vi "UnpoweredState.vi"(8 "error in (no error)":errorcluster, 10 "Cluster in":T2, 11 "Enum in":T1) -> (0 "error out":errorcluster, 2 "Cluster out":T2, 3 "Enum":T1)   [LabVIEW 2018]
uses:
  Type_Def Actuator Controls.ctl
  Type_Def_Current_state_output.ctl
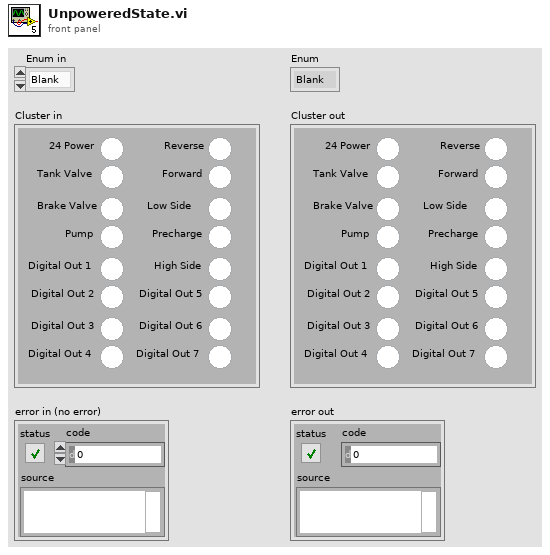
[diagram p1: front panel]
types:
  T1 = typedef "Type_Def_Current_state_output.ctl" = enum16{"Blank", "Systems Check", "Idle", "Ready", "Pushing", "CrawlingPrecharge", "Braking", "Fault", "Boot Up", "Unpowered", "Crawling", "Shutdown", "Service Push", "Service Wait", "Vent", "Precharge", "Cooldown"}
  T2 = typedef "Type_Def Actuator Controls.ctl" = cluster{"Reverse ":bool, "Forward":bool, "Low Side":bool, "Precharge":bool, "High Side":bool, "Digital Out 5":bool, "Digital Out 6":bool, "Digital Out 7 ":bool, "24 Power":bool, "Tank Valve ":bool, "Brake Valve":bool, "Pump":bool, "Digital Out 1 ":bool, "Digital Out 2":bool, "Digital Out 3":bool, "Digital Out 4 ":bool}
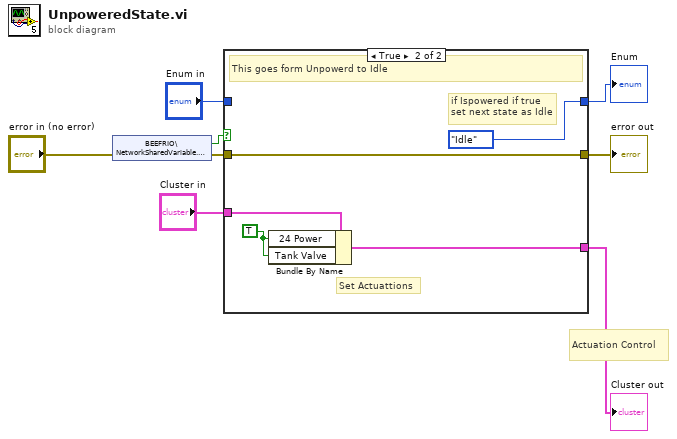
[diagram p0: block diagram]
diagram:
  # "Actuation Control"
  n1 = shared-variable "BEEFRIO\\NetworkSharedVariable.lvlib\\IsPowered"(error in="error in (no error)") -> (w6:bool, error out=w7:errorcluster)
  n2 = case shown="True" w6 {
    tunnel: "Enum in" -> [w11 _]
    tunnel: [w11 Type_Def_Current_state_output."Idle"] -> w2
    tunnel: "Cluster in" -> [w10 w15]
    tunnel: [w10 w14] -> w4
    tunnel: [w9 w13] -> w5
    tunnel: w7 -> [w9 w13]
    frame False {
      # "If isPower is false, then go back to unpowered"
    }
    frame True {
      w12 = TRUE ("Digital Out 5")
      # "if Ispowered if true\nset next state as Idle"
      # "Set Actuattions"
      # "This goes form Unpowerd to Idle"
      n3 = Bundle By Name(cluster=w15, "24 Power"=w12, "Tank Valve"=w12) -> (w14:T2)
    }
  }
  "error out" <- w5
  "Cluster out" <- w4
  "Enum" <- w2
